vi "Waves.vi"(8 "error in (no error) 2":errorcluster caption="错误输入（无错误）", 9 "通道使能引用数组":refnum<vi>[](array[refnum]), 10 "波形图":refnum<vi>, 11 "VISA资源名称输入":refnum<visa-resource-name>) -> (0 "error out 2":errorcluster caption="错误输出", 3 "VISA资源名称输出":refnum<visa-resource-name>)   [LabVIEW 2018]
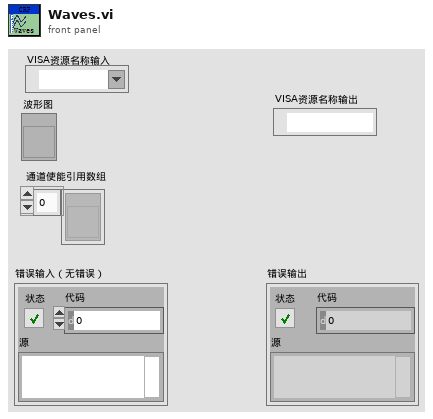
[diagram p1: front panel]
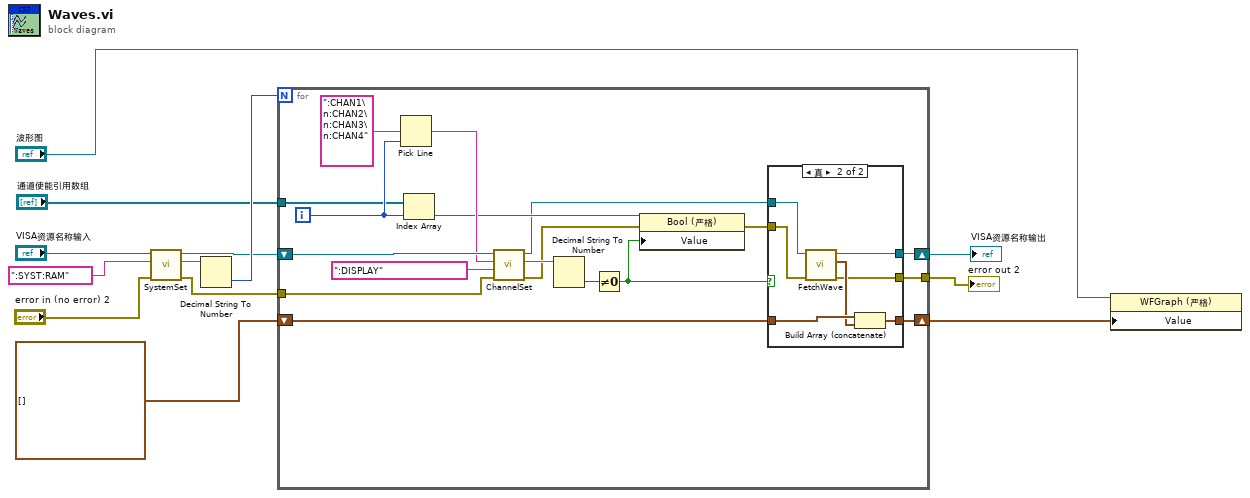
[diagram p0: block diagram]
diagram:
  n1 = call "SystemSet.vi"("error in (no error)"="error in (no error) 2", "SYSTEM命令子系统"=":SYST:RAM", "VISA资源名称"="VISA资源名称输入") -> ("error out"=w7:errorcluster, "查询返回"=w10:string, "VISA资源名称 2"=w8:refnum<visa-resource-name>)  [unwired: 5 in, 1 out]
  n2 = Decimal String To Number(string=w10) -> (number=w9:i32)  [unwired: 2 in, 1 out]
  n3 = for {
    N: w9 -> [_]
    tunnel: w7 -> [w27]
    tunnel: "通道使能引用数组" -> [w24]
    tunnel: [w16] -> w4
    shift-right: [w15] -> w3
    shift-left: w8 -> [w30]
    shift-right: [w17] -> w1
    shift-left: waveform(dbl)[] [] -> [w18]
    i -> [w25]
    n4 = Pick Line(multi-line string=":CHAN1\n:CHAN2\n:CHAN3\n:CHAN4", line index=w25) -> (output string=w28:string)  [unwired: 1 in]
    n5 = Index Array(array=w24, index=w25) -> (element=w23:refnum<vi>)
    n6 = call "ChannelSet.vi"("error in (no error)"=w27, "CHANNLE命令子系统"=":DISPLAY", "通道选择"=w28, "VISA资源名称"=w30) -> ("error out"=w22:errorcluster, "查询返回"=w26:string, "VISA资源名称 2"=w20:refnum<visa-resource-name>)  [unwired: 4 in, 1 out]
    n7 = Decimal String To Number(string=w26) -> (number=w21:i32)  [unwired: 2 in, 1 out]
    n8 = Not Equal To 0?(x=w21) -> (x != 0?=w14:bool)
    n9 = property class="Bool (严格)"(reference=w23, error in=w22, "Value"=w14) -> (error out=w19:errorcluster)  [unwired: 1 out]
    n10 = case shown="真" w14 {
      tunnel: w20 -> [w32 w41]
      tunnel: w19 -> [w33 w40]
      tunnel: w18 -> [w34 w39]
      tunnel: [w34 w37] -> w17
      tunnel: [w33 w36] -> w16
      tunnel: [w32 w35] -> w15
      frame False {
      }
      frame True {
        n11 = call "FetchWave.vi"("error in (no error)"=w40, "VISA资源名称"=w41) -> ("error out"=w36:errorcluster, "波形图"=w38:waveform(dbl), "VISA资源名称 2"=w35:refnum<visa-resource-name>)  [unwired: 7 in]
        n12 = Build Array (concatenate)(w39, w38) -> (w37:waveform(dbl)[])
      }
    }
  }
  "error out 2" <- w4
  "VISA资源名称输出" <- w3
  n13 = property class="WFGraph (严格)"(reference="波形图", "Value"=w1) -> ()  [unwired: 1 in, 2 out]
